vi "SutterTest.vi"() -> ()   [LabVIEW 2012]
panel:
  out "Status command":string
  out "speed 2":i32
  out "word swapped 4":i32
  out "speed":i32
  out "word swapped 2":i32
  out "word swapped":i32
  out "String":string
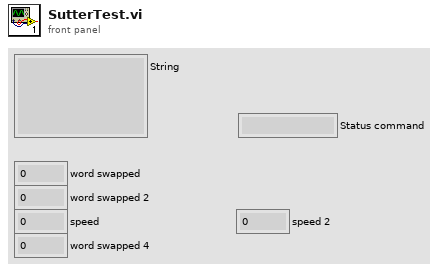
[diagram p1: front panel]
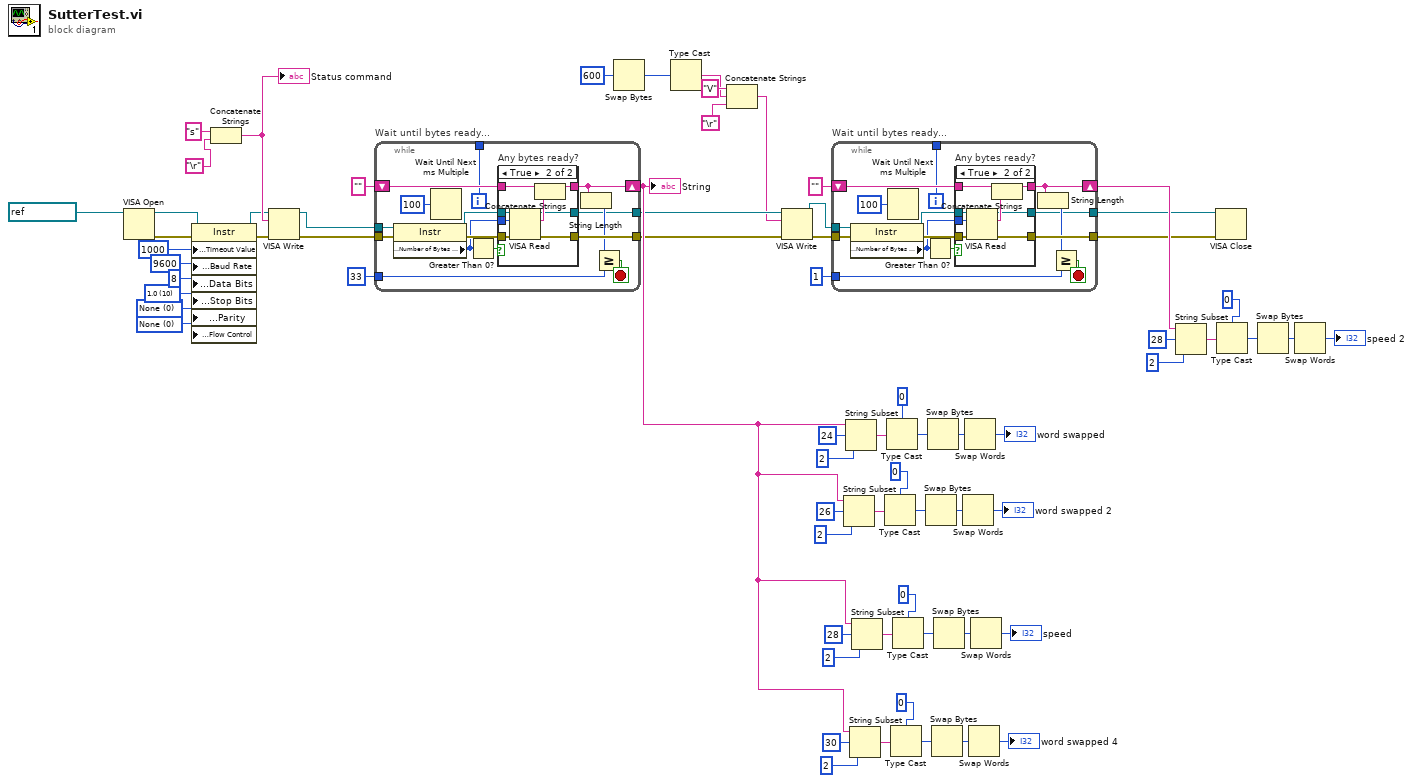
[diagram p0: block diagram]
diagram:
  w61 = u16 0 items=["None", "XON/XOFF", "RTS/CTS", "XON/XOFF & RTS/CTS", "DTR/DSR", "XON/XOFF & DTR/DSR"] ("Serial Settings:Flow Control")
  w60 = u16 0 items=["None", "Odd", "Even", "Mark", "Space"] ("Serial Settings:Parity")
  w59 = u16 10 items=["1.0"=10, "1.5"=15, "2.0"=20] ("Serial Settings:Stop Bits")
  n1 = VISA Open(VISA resource name=refnum<visa-resource-name> "COM10") -> (VISA resource name=w56:refnum<visa-resource-name>, error out=w53:errorcluster)  [unwired: 4 in]
  n2 = property on="Property Node" class="Instr"(reference=w56, error in=w53, "General Settings:Timeout Value"=u32 1000, "Serial Settings:Baud Rate"=u32 9600, "Serial Settings:Data Bits"=u16 8, "Serial Settings:Stop Bits"=w59, "Serial Settings:Parity"=w60, "Serial Settings:Flow Control"=w61) -> (reference out=w54:refnum<visa-resource-name>, error out=w52:errorcluster)
  n3 = Concatenate Strings("s" ("string"), "\r") -> (w66:string)
  "Status command" <- w66
  n4 = VISA Write(VISA resource name=w54, write buffer=w66, error in (no error)=w52) -> (VISA resource name out=w65:refnum<visa-resource-name>, error out=w64:errorcluster)  [unwired: 1 out]
  n5 = while "Wait until bytes ready..." {
    tunnel: w65 -> [w84]
    tunnel: w64 -> [w83]
    tunnel: [w79] -> w15
    tunnel: 33 ("bytes to read") -> [w75]
    shift-right: [w77] -> w23
    shift-left: "" -> [w78]
    tunnel: [w71] -> _
    tunnel: [w70] -> w17
    i -> [w71]
    stop <- w74 stop-if-true
    n6 = property class="Instr"(reference=w84, error in=w83) -> (reference out=w80:refnum<visa-resource-name>, error out=w81:errorcluster, "Serial Settings:Number of Bytes at Serial Port"=w72:u32)
    n7 = Wait Until Next ms Multiple(millisecond multiple=u32 100) -> ()  [unwired: 1 out]
    n8 = Greater Than 0?(x=w72) -> (x > 0?=w73:bool)
    n9 = case "Any bytes ready?" shown="True" w73 {
      tunnel: w81 -> [w87 w95]
      tunnel: w80 -> [w85 w94]
      tunnel: [w87 w93] -> w79
      tunnel: w78 -> [w86 w92]
      tunnel: [w86 w90] -> w77
      tunnel: w72 -> [_ w89]
      tunnel: [w85 w88] -> w70
      frame False {
      }
      frame True {
        n10 = VISA Read(VISA resource name=w94, byte count=w89, error in (no error)=w95) -> (VISA resource name out=w88:refnum<visa-resource-name>, read buffer=w91:string, error out=w93:errorcluster)  [unwired: 1 out]
        n11 = Concatenate Strings(w92, w91) -> (w90:string)
      }
    }
    n12 = String Length(string=w77) -> (length=w76:i32)
    n13 = Greater Or Equal?(x=w76, y=w75) -> (x >= y?=w74:bool)
  }
  "String" <- w23
  n14 = Swap Bytes(anything=u16 600 ("data")) -> (byte swapped=w22:u16)
  n15 = Type Cast(x=w22) -> (*(type *) &x=w18:string)  [unwired: 1 out]
  n16 = Concatenate Strings("V" ("string"), w18, "\r") -> (w16:string)
  n17 = VISA Write(VISA resource name=w17, write buffer=w16, error in (no error)=w15) -> (VISA resource name out=w11:refnum<visa-resource-name>, error out=w12:errorcluster)  [unwired: 1 out]
  n18 = while "Wait until bytes ready..." {
    tunnel: w11 -> [w110]
    tunnel: w12 -> [w109]
    tunnel: [w105] -> w1
    tunnel: 1 ("bytes to read") -> [w101]
    shift-right: [w103] -> w3
    shift-left: "" -> [w104]
    tunnel: [w97] -> _
    tunnel: [w96] -> w2
    i -> [w97]
    stop <- w100 stop-if-true
    n19 = property class="Instr"(reference=w110, error in=w109) -> (reference out=w106:refnum<visa-resource-name>, error out=w107:errorcluster, "Serial Settings:Number of Bytes at Serial Port"=w98:u32)
    n20 = Wait Until Next ms Multiple(millisecond multiple=u32 100) -> ()  [unwired: 1 out]
    n21 = Greater Than 0?(x=w98) -> (x > 0?=w99:bool)
    n22 = case "Any bytes ready?" shown="True" w99 {
      tunnel: w107 -> [w113 w121]
      tunnel: w106 -> [w111 w120]
      tunnel: [w113 w119] -> w105
      tunnel: w104 -> [w112 w118]
      tunnel: [w112 w116] -> w103
      tunnel: w98 -> [_ w115]
      tunnel: [w111 w114] -> w96
      frame False {
      }
      frame True {
        n23 = VISA Read(VISA resource name=w120, byte count=w115, error in (no error)=w121) -> (VISA resource name out=w114:refnum<visa-resource-name>, read buffer=w117:string, error out=w119:errorcluster)  [unwired: 1 out]
        n24 = Concatenate Strings(w118, w117) -> (w116:string)
      }
    }
    n25 = String Length(string=w103) -> (length=w102:i32)
    n26 = Greater Or Equal?(x=w102, y=w101) -> (x >= y?=w100:bool)
  }
  n27 = String Subset(string=w23, offset (0)=26, length (rest)=2 ("length (rest)")) -> (substring=w42:string)
  n28 = String Subset(string=w23, offset (0)=24, length (rest)=2 ("length (rest)")) -> (substring=w49:string)
  n29 = String Subset(string=w23, offset (0)=30, length (rest)=2 ("length (rest)")) -> (substring=w28:string)
  n30 = String Subset(string=w23, offset (0)=28, length (rest)=2 ("length (rest)")) -> (substring=w35:string)
  n31 = Type Cast(type=0, x=w42) -> (*(type *) &x=w43:i32)
  n32 = Type Cast(type=0, x=w49) -> (*(type *) &x=w50:i32)
  n33 = Type Cast(type=0, x=w28) -> (*(type *) &x=w29:i32)
  n34 = Type Cast(type=0, x=w35) -> (*(type *) &x=w36:i32)
  n35 = Swap Bytes(anything=w43) -> (byte swapped=w44:i32)
  n36 = Swap Bytes(anything=w50) -> (byte swapped=w51:i32)
  n37 = Swap Bytes(anything=w29) -> (byte swapped=w30:i32)
  n38 = Swap Bytes(anything=w36) -> (byte swapped=w37:i32)
  n39 = Swap Words(1:w44) -> (0:→"word swapped 2":i32)
  n40 = Swap Words(1:w51) -> (0:→"word swapped":i32)
  n41 = Swap Words(1:w30) -> (0:→"word swapped 4":i32)
  n42 = Swap Words(1:w37) -> (0:→"speed":i32)
  n43 = String Subset(string=w3, offset (0)=28, length (rest)=2 ("length (rest)")) -> (substring=w8:string)
  n44 = VISA Close(VISA resource name=w2, error in (no error)=w1) -> ()  [unwired: 1 out]
  n45 = Type Cast(type=0, x=w8) -> (*(type *) &x=w9:i32)
  n46 = Swap Bytes(anything=w9) -> (byte swapped=w10:i32)
  n47 = Swap Words(1:w10) -> (0:→"speed 2":i32)
